vi "Washer HCC Newfi Main.vi"() -> ()   [LabVIEW 2012]
uses:
  Nufi/Newfi LDN/Washer.ctl
  Nufi/Newfi LDN/Washer Details.ctl
  Nufi/Newfi LDN/Unit Type.ctl
  <vilib>/Utility/file.llb/Read From Spreadsheet File (string).vi
  Drivers/Agilent 34970/Agilent 34970.lvlib
panel:
  in  "Tab Control 3":enum32{"Debug Info"}(tab)
  out "Agilent Channels DAQ":string
  out "Current":dbl[](array[numeric])
  out "States Out":string
  out "States Out 2":string
  out "Save Array":bool[](array[boolean])
  out "Board Index.":i32[](array[numeric])
  out "error out":errorcluster
  in  "error in (no error)":errorcluster
  in  "Tab Control 2":enum32{"Page 1"}(tab)
  in  "Quit":bool
  out "Timer 2":dbl format="%<%H:%M:%S>t"
  in  "Connected Board ID's (Newfi)":string[](array[string])
  in  "Board Index":i32[](array[numeric])
  in  "Back Button":bool
  in  "Settings":bool
  out "Description":string="Application Title"
  out "Waveform Chart":dbl(graph)
  in  "Open Panel":T1 {"Unit Type" items=["", "Viper", "Hawk", "Other"]; "Current" format="%.2f"; "Day Cycle Count" format="%04d"}
  in  "Tab Control":enum32{"Page 1", "Page 2"}(tab)
  in  "Array 4":T1[](array[typedef]) {"Unit Type" items=["", "Viper", "Hawk", "Other"]; "Current" format="%.2f"; "Day Cycle Count" format="%04d"}
  in  "Array 3":T1[](array[typedef]) {"Unit Type" items=["", "Viper", "Hawk", "Other"]; "Current" format="%.2f"; "Day Cycle Count" format="%04d"}
  in  "Array":T1[](array[typedef]) {"Unit Type" items=["", "Viper", "Hawk", "Other"]; "Current" format="%.2f"; "Day Cycle Count" format="%04d"}
  in  "Array 2":T1[](array[typedef]) {"Unit Type" items=["", "Viper", "Hawk", "Other"]; "Current" format="%.2f"; "Day Cycle Count" format="%04d"}
  out "Collecting Agilent Data":bool
  in  "Agilent Scan Rate (Seconds)":i32=5
  in  "Status Output Locations":path[](array[path])
  in  "Configuration Path":path=path "C:/Newfi Exe/Newfi Exe Locations.ini"
  out "Time":string="Settings"
  in  "Station and Board IDs":path=path "C:/Newfi Exe/Stations and Board IDs.ini"
  in  "Agilent":refnum<visa-resource-name>="AGILENT_HCC"
  in  "Start DAQ Loop":bool
  # "Washer HCC"
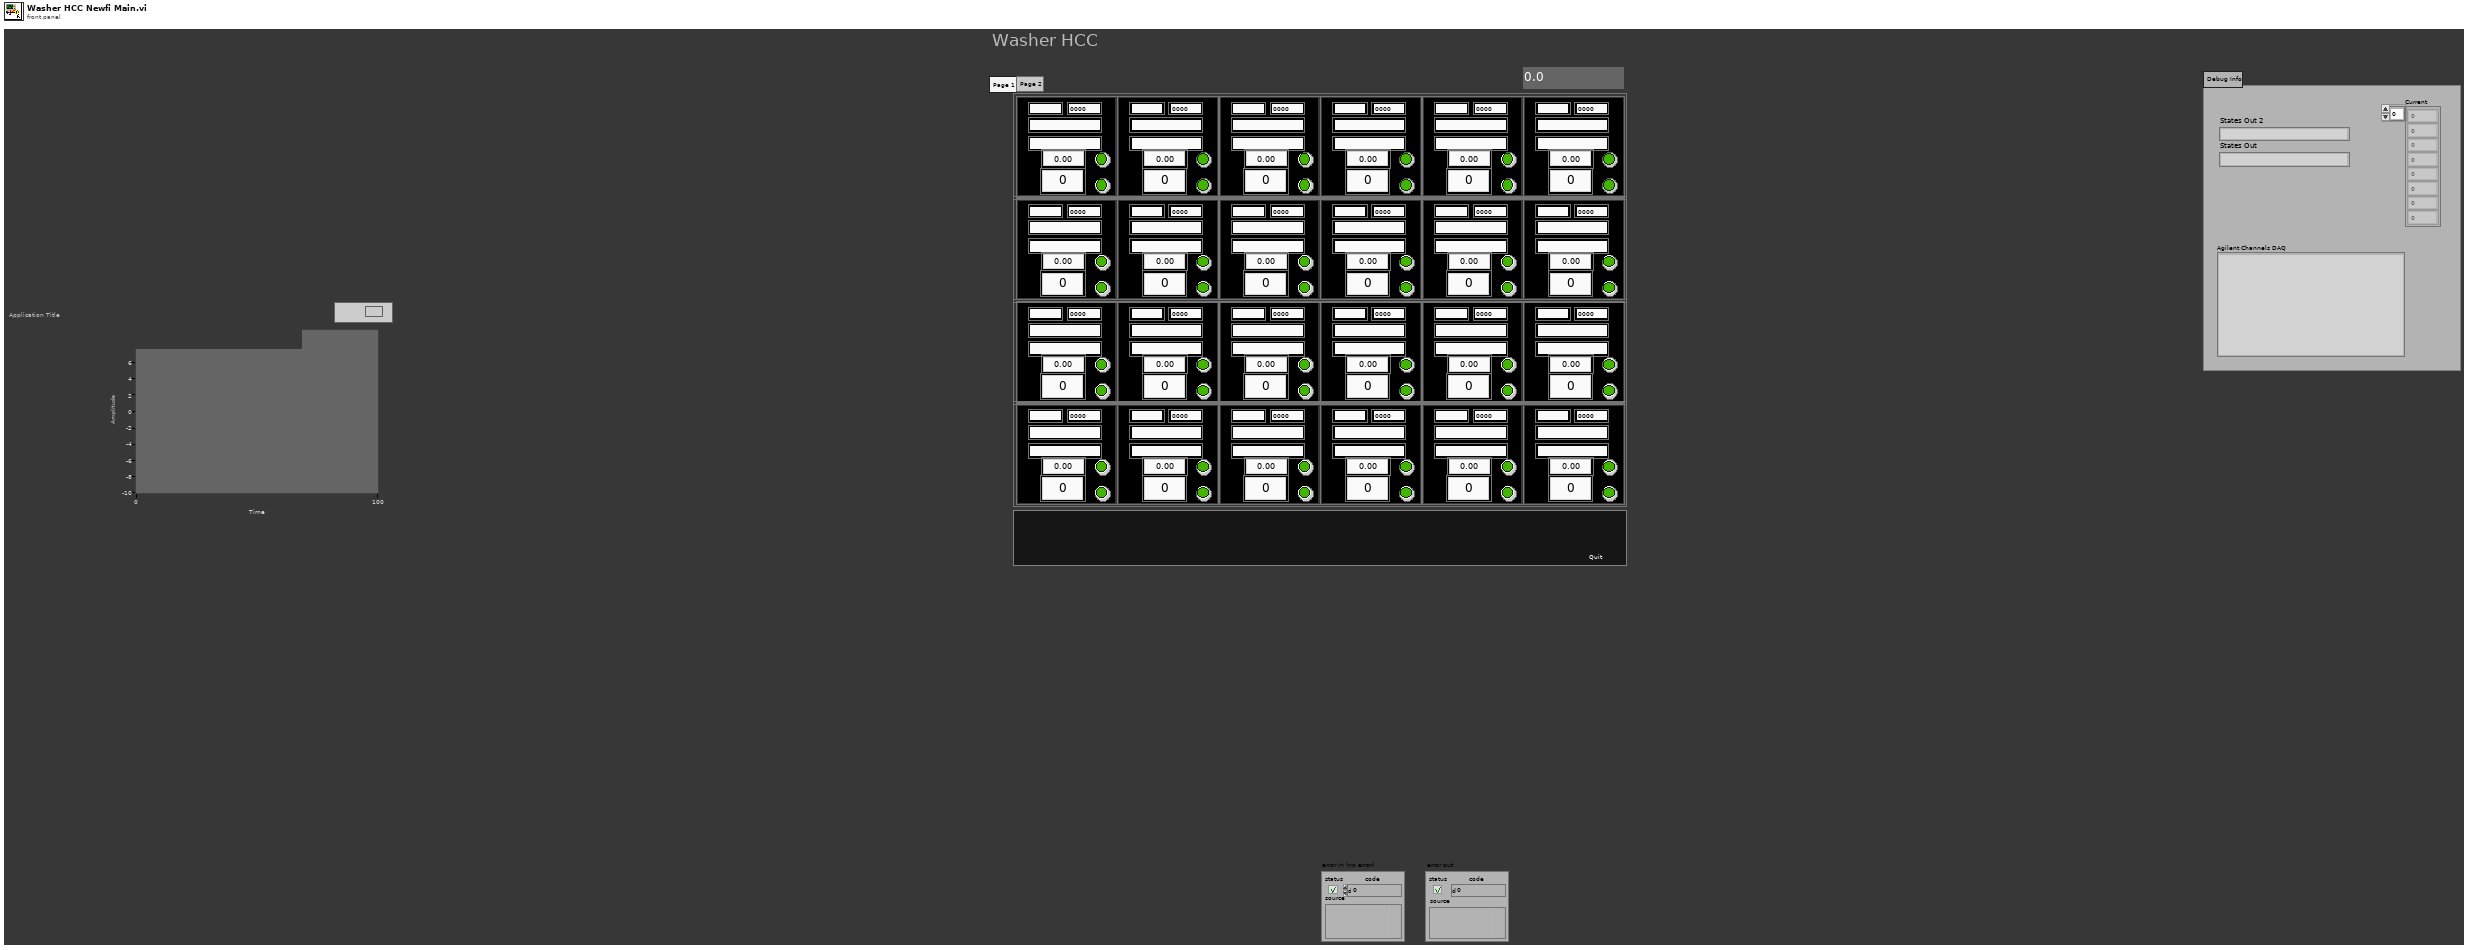
[diagram p1: front panel]
types:
  T1 = typedef "Washer.ctl" = cluster{"Serial Number":string, "Day Cycle Count":i32, "Station Label":string, "Status Color":u32, "Current Run Start Time":dbl, "Audit Alert":bool, "Washer Details":T2, "Board ID":string, "Boolean":bool, "RPM":u32, "Current":dbl, "Current Path":path, "Saving":bool, "Unit Type":T3}
  T2 = typedef "Washer Details.ctl" = cluster{"Cycle Count":string, "Status":string, "Notes":string, "Lab ID":string, "Total Time On":string, "TR Number":string}
  T3 = typedef "Unit Type.ctl" = u32
  T4 = enum16{"4 1/2", "5 1/2", "6 1/2", "Least", "Highest", "Default"}
  T5 = enum16{"100 mV", "1 V", "10 V", "100 V", "300 V", "Auto", "Minimum", "Maximum"}
  T6 = cluster{"Agilent":refnum<visa-resource-name>, "Agilent Scan Rate (Seconds)":i32, "Current":dbl[]}
  T7 = enum32{"invalid app kind", "Development System", "Run Time System", "Student Edition", "Embedded LabVIEW", "Evaluation", "Custom"}
  T8 = cluster{"Current VI Reference":refnum<vi>, "Close Panel on Exit?":bool}
  T9 = enum32{"Invalid", "Standard", "Closed", "Hidden", "Minimized", "Maximized"}
  T10 = cluster{"Core":cluster{"Current VI Reference":refnum<vi>, "Close Panel on Exit?":bool}, "Array":T1[], "Array 2":T1[], "Status Output Locations":path[], "Open Panel":T1, "Array 3":T1[], "Array 4":T1[], "Board Index":i32[], "Connected Board ID's (Newfi)":string[], "Agilent Channels":string, "Start DAQ Loop":bool, "Log Debug":string[], "Log Inv & MC":string[], "Station IDs":string[], "Last Save Time":string}
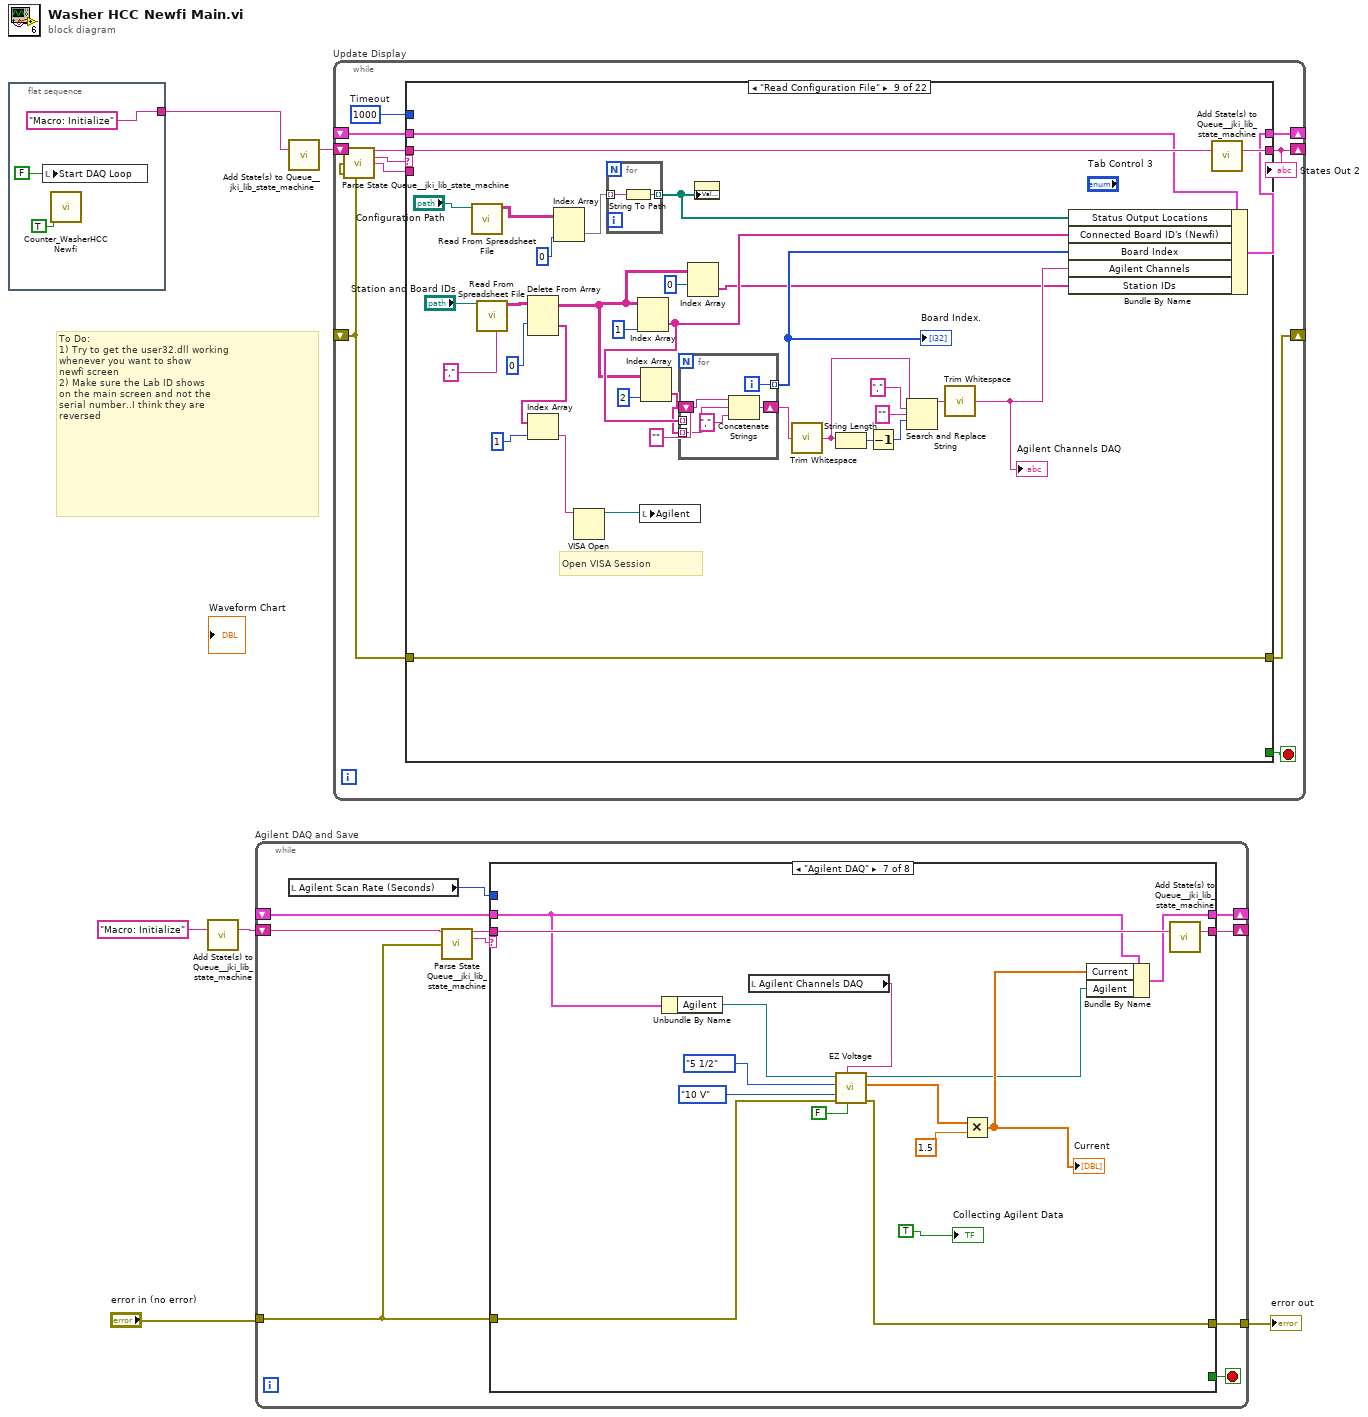
[diagram p0: block diagram]
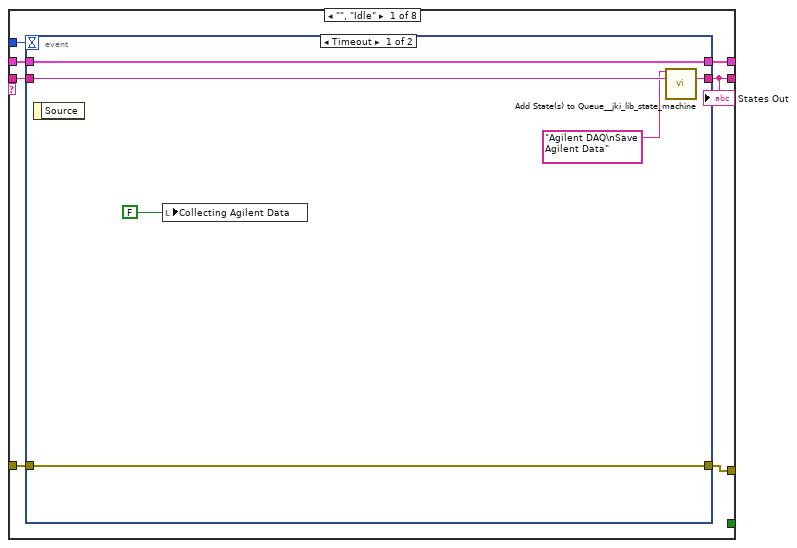
[diagram p2: hidden frame]
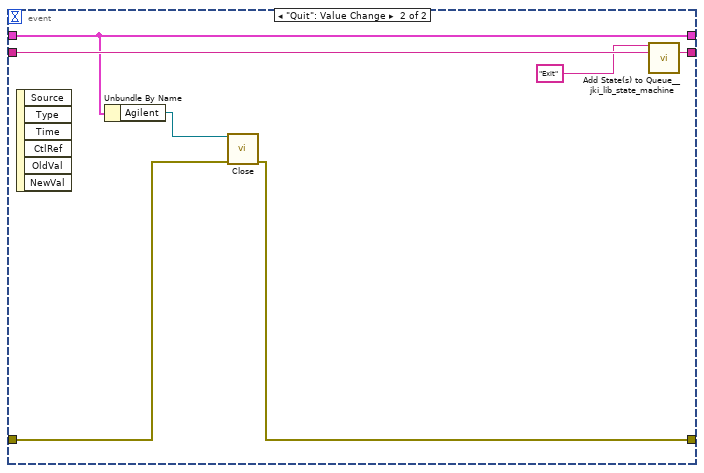
[diagram p3: hidden frame]
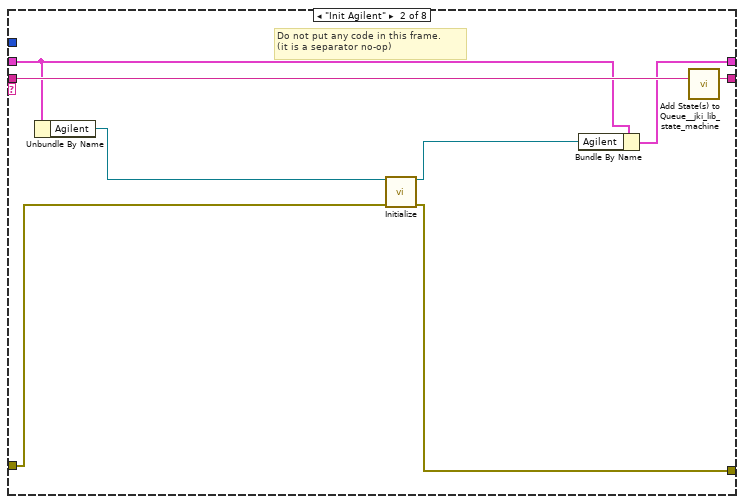
[diagram p4: hidden frame]
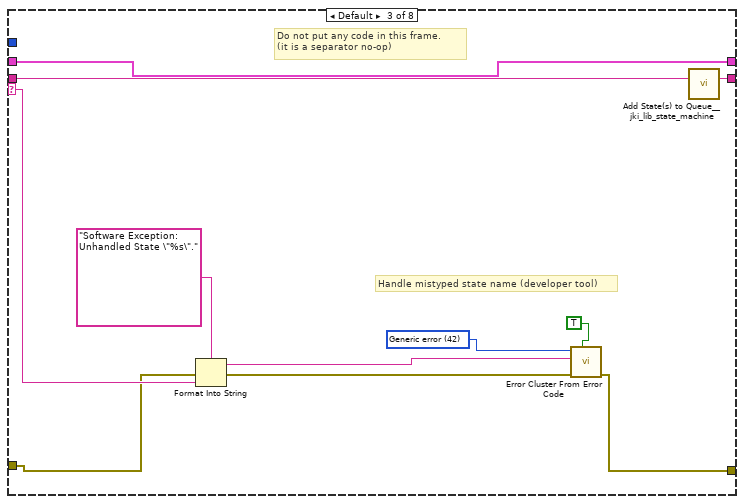
[diagram p5: hidden frame]
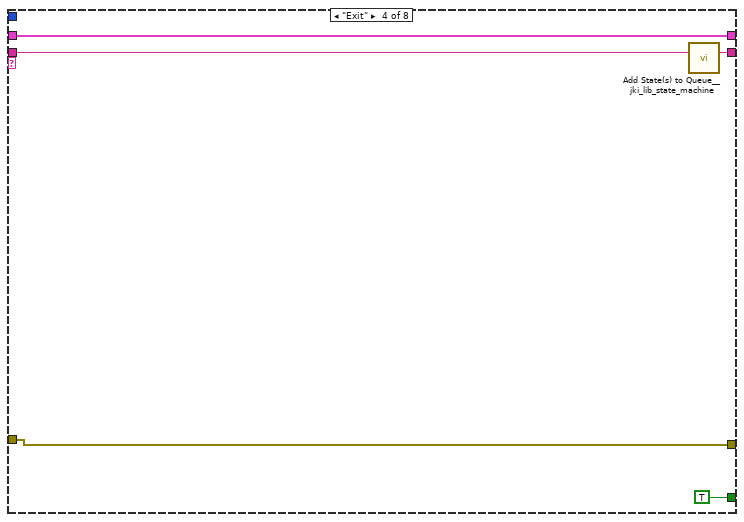
[diagram p6: hidden frame]
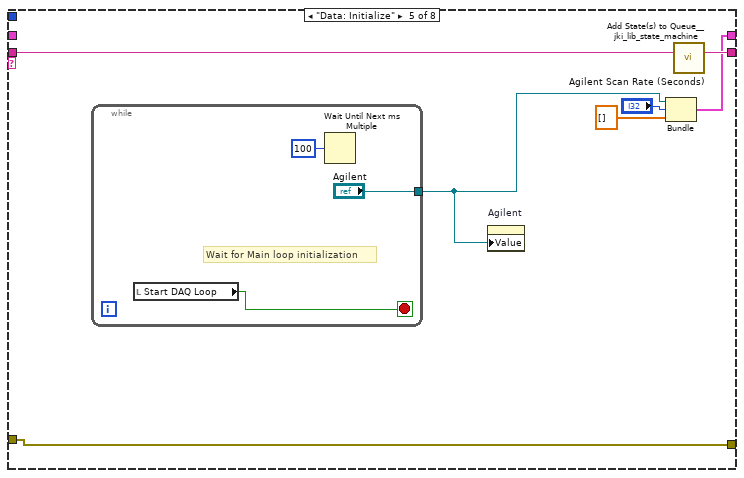
[diagram p7: hidden frame]
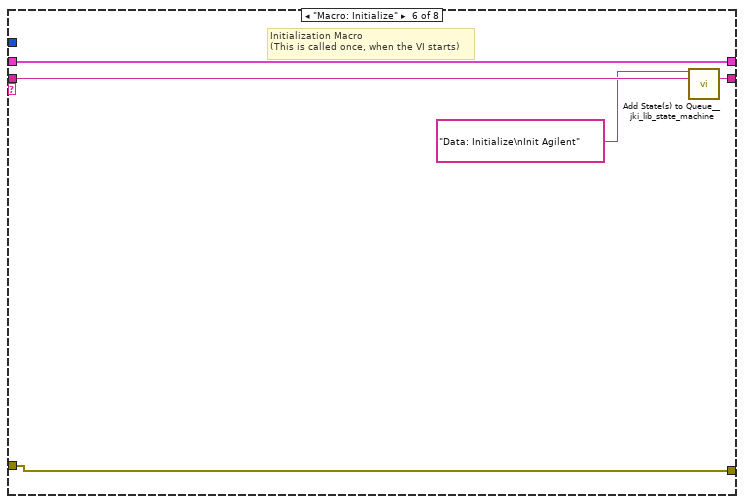
[diagram p8: hidden frame]
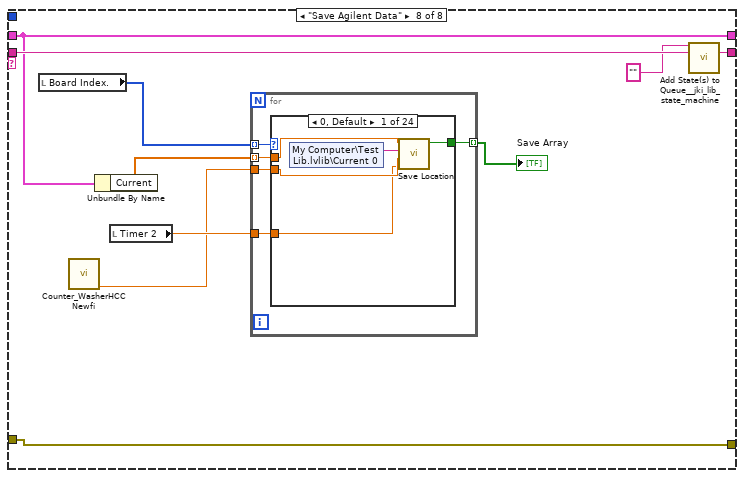
[diagram p9: hidden frame]
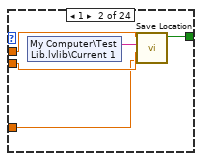
[diagram p10: hidden frame]
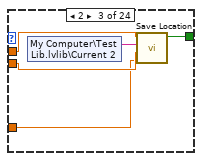
[diagram p11: hidden frame]
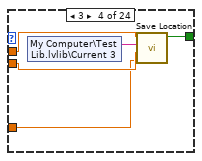
[diagram p12: hidden frame]
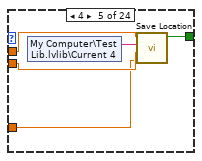
[diagram p13: hidden frame]
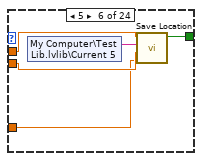
[diagram p14: hidden frame]
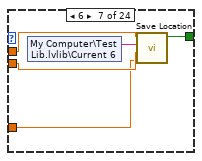
[diagram p15: hidden frame]
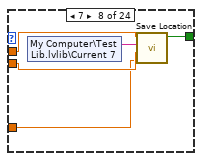
[diagram p16: hidden frame]
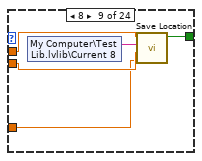
[diagram p17: hidden frame]
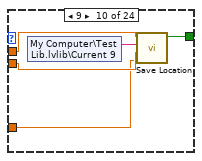
[diagram p18: hidden frame]
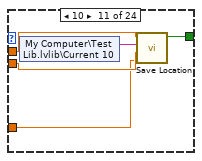
[diagram p19: hidden frame]
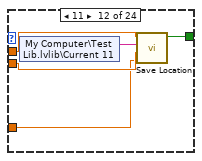
[diagram p20: hidden frame]
diagram:
  # "To Do:\n1) Try to get the user32.dll working\nwhenever you want to show\nnewfi screen\n2) Make sure the Lab ID shows\non the main screen and not the \nserial number..I think they are \nreversed"
  n1 = flat-sequence {
    tunnel: ["Macro: Initialize"] -> w3
    frame #0 {
      n2 = local write "Start DAQ Loop"(FALSE ("Start DAQ Loop")) -> ()
      n3 = call "Counter_WasherHCC Newfi.vi"("Reset"=TRUE) -> ()  [unwired: 10 in, 1 out]
    }
  }
  n4 = call <vilib>:"Add State(s) to Queue__jki_lib_state_machine.vi"("State(s) in (\"\")"="Macro: Initialize") -> ("States Out"=w2:string)  [unwired: 14 in]
  n5 = while "Agilent DAQ and Save" {
    shift-right: [w14] -> _
    shift-left: _ -> [w13]
    shift-right: [w16] -> _
    shift-left: w2 -> [w17]
    tunnel: "error in (no error)" -> [w10]
    tunnel: [w12] -> w5
    stop <- w15 stop-if-true
    n6 = local read "Agilent Scan Rate (Seconds)"() -> (w11:i32)
    n7 = call <vilib>:"Parse State Queue__jki_lib_state_machine.vi"("State Queue"=w17, "Error In (no error)"=w10) -> ("Remaining States"=w18:string, "Current State"=w19:string)  [unwired: 11 in, 1 out]
    n8 = case shown="\"Agilent DAQ\"" w19 {
      selector: w19 -> [_ _ w50 _ _ _ _ _]
      tunnel: w18 -> [w26 w47 w58 w63 w70 w78 w94 w104]
      tunnel: w13 -> [w24 w44 w56 w61 _ w76 w84 w98]
      tunnel: [w25 w46 w57 w62 w69 w77 w93 w103] -> w16
      tunnel: [_ _ _ TRUE _ _ _ _] -> w15
      tunnel: [w23 w43 w56 w61 w68 w76 w83 w98] -> w14
      tunnel: w11 -> [w22 _ _ _ _ _ _ _]
      tunnel: w10 -> [w21 w41 w49 w59 w65 w74 w86 w102]
      tunnel: [w20 w40 w48 w59 w65 w74 w85 w102] -> w12
      frame "", "Idle" {
        n9 = event shown="[0] Timeout" {
          selector: _ -> [_ _]
          dyn-events: _ -> [_ _]
          timeout: w22 -> [_ _]
          tunnel: w26 -> [w32 w39]
          tunnel: [w31 w38] -> w25
          tunnel: w24 -> [w30 w36]
          tunnel: [w30 w36] -> w23
          tunnel: [w27 w33] -> w20
          tunnel: w21 -> [w27 w34]
          event Timeout {
            n10 = event-data() -> ()  [unwired: 1 in, 1 out]
            n11 = local write "Collecting Agilent Data"(FALSE ("Collecting Agilent Data")) -> ()
            n12 = call <vilib>:"Add State(s) to Queue__jki_lib_state_machine.vi"("State(s) in Front (\"\")"="Agilent DAQ\nSave Agilent Data", "State(s) in (\"\")"=w32) -> ("States Out"=w31:string)  [unwired: 13 in]
          }
          event "Quit": Value Change {
            n13 = event-data() -> ()  [unwired: 1 in, 6 out]
            n14 = Unbundle By Name(w36) -> ("Agilent"=w35:refnum<visa-resource-name>)
            n15 = call "Close.vi"("VISA Resource Name"=w35, "error in (no error)"=w34) -> ("error out"=w33:errorcluster)  [unwired: 13 in]
            n16 = call <vilib>:"Add State(s) to Queue__jki_lib_state_machine.vi"("State(s) in Front (\"\")"="Exit", "State(s) in (\"\")"=w39) -> ("States Out"=w38:string)  [unwired: 13 in]
          }
        }
        "States Out" <- w25
      }
      frame "Init Agilent" {
        # "Do not put any code in this frame.\n(it is a separator no-op)"
        n17 = Unbundle By Name(w44) -> ("Agilent"=w45:refnum<visa-resource-name>)
        n18 = call "Initialize.vi"("VISA Resource Name"=w45, "error in (no error)"=w41) -> ("VISA Resource Name Out"=w42:refnum<visa-resource-name>, "error out"=w40:errorcluster)  [unwired: 12 in]
        n19 = Bundle By Name(cluster=w44, "Agilent"=w42) -> (w43:T6)
        n20 = call <vilib>:"Add State(s) to Queue__jki_lib_state_machine.vi"("State(s) in (\"\")"=w47) -> ("States Out"=w46:string)  [unwired: 14 in]
      }
      frame Default {
        w52 = 42 items=["No error", "Argument error", "Memory is full", "Out of zone", "End of file", "File already open", "Generic file I/O error", "File not found", "File permission error", "Disk is full", "Duplicate path", "Too many files open", "System feature not enabled", "Resource file not found", "Cannot add resource", "Resource not found", "Image not found", "Image memory error", "Pen does not exist", "Config type invalid", "Config token not found", "Config parse error", "Config memory error", "Bad external code format", "Bad external code offset", "External code not present", "Null window", "Destroy window error", "Null menu", "Print aborted", "Bad print record", "Print driver error", "Windows error during printing", "Memory error during printing", "Print dialog error", "Generic print error", "Invalid device refnum", "Device not found", "Device parameter error", "Device unit error", "Cannot open device", "Device call aborted", "Generic error", "Cancelled by user", "Object ID too low", "Object ID too high", "Object not in heap", "Unknown heap", "Unknown object (invalid DefProc)", "Unknown object (DefProc not in table)", "Message out of range", "Invalid (null) method", "Unknown message", "Manager call not supported", "Bad address", "Network operation in progress", "Network operation timed out", "Connection is busy", "Network attribute not supported", "Network error", "Address in use", "System out of memory", "Connection aborted", "Connection refused", "Not connected", "Already connected", "Connection closed", "Initialization error (interapplication manager)", "Bad occurrence", "Wait on unbound occurrence handler", "Occurrence queue overflow", "Datalog type conflict", "Unused", "Unrecognized type (interapplication manager)", "Memory corrupt", "Failed to make temporary DLL", "Old CIN version", "Drag socket not found", "Failed to load drop-object", "Failed to register OLE object", "Failed to release OLE object", "Format specifier type mismatch", "Unknown format specifier", "Too few format specifiers", "Too many format specifiers", "Scan failed", "Newer CIN version", "Error converting to variant", "Runtime menu error", "Password tampered", "Variant attribute not found", "Incompatible variant data type", "Event data is not available", "Event Store is not present", "Occurrence is not found", "Event Queue is not created", "Event info is not available", "Refnum passed is NULL", "Error retrieving Class GUID", "Error retrieving CoClass GUID", "Error retrieving TypeLib GUID.", "Bad built application magic bytes.", "Specific driver is different from the specific driver associated with the Logical Name.", "There is no session opened to the class driver.", "Max Error", "MAX - Error with config objects", "MAX - Error loading configuration", "MAX - Group not supported"]
        # "Handle mistyped state name (developer tool)"
        # "Do not put any code in this frame.\n(it is a separator no-op)"
        n21 = Format Into String(format string="Software Exception: Unhandled State \"%s\"." ("message"), error in=w49, w50) -> (resulting string=w53:string, error out=w54:errorcluster)  [unwired: 1 in]
        n22 = call <vilib>:"Error Cluster From Error Code.vi"("show call chain? (False)"=TRUE, "error in (no error)"=w54, "error message (\"\")"=w53, "error code (0)"=w52) -> ("error out"=w48:errorcluster)  [unwired: 5 in]
        n23 = call <vilib>:"Add State(s) to Queue__jki_lib_state_machine.vi"("State(s) in (\"\")"=w58) -> ("States Out"=w57:string)  [unwired: 14 in]
      }
      frame "Exit" {
        n24 = call <vilib>:"Add State(s) to Queue__jki_lib_state_machine.vi"("State(s) in (\"\")"=w63) -> ("States Out"=w62:string)  [unwired: 14 in]
      }
      frame "Data: Initialize" {
        n25 = while {
          tunnel: ["Agilent"] -> w64
          stop <- w72 stop-if-true
          # "Wait for Main loop initialization"
          n26 = local read "Start DAQ Loop"() -> (w72:bool)
          n27 = Wait Until Next ms Multiple(millisecond multiple=u32 100) -> ()  [unwired: 1 out]
        }
        n28 = property on="Agilent" class="VISAName"("Value"=w64) -> ()  [unwired: 2 in, 2 out]
        n29 = Bundle("Agilent"=w64, "Agilent Scan Rate (Seconds)"="Agilent Scan Rate (Seconds)", "Current"=dbl[] []) -> (w68:T6)  [unwired: 1 in]
        n30 = call <vilib>:"Add State(s) to Queue__jki_lib_state_machine.vi"("State(s) in (\"\")"=w70) -> ("States Out"=w69:string)  [unwired: 14 in]
      }
      frame "Macro: Initialize" {
        # "Initialization Macro\n(This is called once, when the VI starts)"
        n31 = call <vilib>:"Add State(s) to Queue__jki_lib_state_machine.vi"("State(s) in Front (\"\")"="Data: Initialize\nInit Agilent", "State(s) in (\"\")"=w78) -> ("States Out"=w77:string)  [unwired: 13 in]
      }
      frame "Agilent DAQ" {
        n32 = Unbundle By Name(w84) -> ("Agilent"=w92:refnum<visa-resource-name>)
        n33 = local read "Agilent Channels DAQ"() -> (w81:string)
        n34 = call "EZ Voltage.vi"("AC/DC (F:DC)"=FALSE, "Scan List (empty)"=w81, "error in (no error)"=w86, "Range (5:Auto)"=T5."10 V", "Resolution (5:Default)"=T4."5 1/2", "VISA Resource Name"=w92) -> ("error out"=w85:errorcluster, "Output Array"=w88:dbl[], "VISA Resource Name Out"=w79:refnum<visa-resource-name>)  [unwired: 3 in]
        n35 = Multiply(x=w88, y=1.5) -> (x*y=w80:dbl[])
        "Current" <- w80
        n36 = Bundle By Name(cluster=w84, "Current"=w80, "Agilent"=w79) -> (w83:T6)
        n37 = call <vilib>:"Add State(s) to Queue__jki_lib_state_machine.vi"("State(s) in (\"\")"=w94) -> ("States Out"=w93:string)  [unwired: 14 in]
        "Collecting Agilent Data" <- TRUE
      }
      frame "Save Agilent Data" {
        n38 = local read "Board Index."() -> (w99:i32[])
        n39 = call "Counter_WasherHCC Newfi.vi"() -> ("Count"=w96:dbl)  [unwired: 11 in]
        n40 = Unbundle By Name(w98) -> ("Current"=w101:dbl[])
        n41 = local read "Timer 2"() -> (w97:dbl)
        n42 = for {
          tunnel: w99 -> [w109] mode=indexing
          tunnel: w101 -> [w108] mode=indexing
          tunnel: w96 -> [w107]
          tunnel: [w106] -> w100 mode=indexing
          tunnel: w97 -> [w105]
          n43 = case shown="0, Default" w109 {
            tunnel: w108 -> [w113 w118 w123 w128 w133 w138 w143 w149 w153 w158 w164 w168 w174 w178 w183 w188 w193 w198 w203 w208 w213 w218 w224 w226]
            tunnel: w107 -> [w112 w117 w122 w127 w132 w137 w142 w147 w152 w157 w162 w167 w172 w177 w182 w187 w192 w197 w202 w207 w212 w217 w222 w228]
            tunnel: [w111 w116 w121 w126 w131 w136 w141 w146 w151 w156 w161 w166 w171 w176 w181 w186 w191 w196 w201 w206 w211 w216 w221 w227] -> w106
            tunnel: w105 -> [w110 w115 w120 w125 w130 w135 w140 w145 w150 w155 w160 w165 w170 w175 w180 w185 w190 w195 w200 w205 w210 w215 w220 w225]
            frame 0, Default {
              n44 = shared-variable "My Computer\\Test Lib.lvlib\\Current 0"() -> (w114:string)  [unwired: 1 in, 1 out]
              n45 = call "Save Location.vi"("Timer Seconds"=w110, "Counter"=w112, "String"=w114, "Current"=w113) -> ("Saving"=w111:bool)  [unwired: 7 in]
            }
            frame 1 {
              n46 = shared-variable "My Computer\\Test Lib.lvlib\\Current 1"() -> (w119:string)  [unwired: 1 in, 1 out]
              n47 = call "Save Location.vi"("Timer Seconds"=w115, "Counter"=w117, "String"=w119, "Current"=w118) -> ("Saving"=w116:bool)  [unwired: 7 in]
            }
            frame 2 {
              n48 = shared-variable "My Computer\\Test Lib.lvlib\\Current 2"() -> (w124:string)  [unwired: 1 in, 1 out]
              n49 = call "Save Location.vi"("Timer Seconds"=w120, "Counter"=w122, "String"=w124, "Current"=w123) -> ("Saving"=w121:bool)  [unwired: 7 in]
            }
            frame 3 {
              n50 = shared-variable "My Computer\\Test Lib.lvlib\\Current 3"() -> (w129:string)  [unwired: 1 in, 1 out]
              n51 = call "Save Location.vi"("Timer Seconds"=w125, "Counter"=w127, "String"=w129, "Current"=w128) -> ("Saving"=w126:bool)  [unwired: 7 in]
            }
            frame 4 {
              n52 = shared-variable "My Computer\\Test Lib.lvlib\\Current 4"() -> (w134:string)  [unwired: 1 in, 1 out]
              n53 = call "Save Location.vi"("Timer Seconds"=w130, "Counter"=w132, "String"=w134, "Current"=w133) -> ("Saving"=w131:bool)  [unwired: 7 in]
            }
            frame 5 {
              n54 = shared-variable "My Computer\\Test Lib.lvlib\\Current 5"() -> (w139:string)  [unwired: 1 in, 1 out]
              n55 = call "Save Location.vi"("Timer Seconds"=w135, "Counter"=w137, "String"=w139, "Current"=w138) -> ("Saving"=w136:bool)  [unwired: 7 in]
            }
            frame 6 {
              n56 = shared-variable "My Computer\\Test Lib.lvlib\\Current 6"() -> (w144:string)  [unwired: 1 in, 1 out]
              n57 = call "Save Location.vi"("Timer Seconds"=w140, "Counter"=w142, "String"=w144, "Current"=w143) -> ("Saving"=w141:bool)  [unwired: 7 in]
            }
            frame 7 {
              n58 = shared-variable "My Computer\\Test Lib.lvlib\\Current 7"() -> (w148:string)  [unwired: 1 in, 1 out]
              n59 = call "Save Location.vi"("Timer Seconds"=w145, "Counter"=w147, "String"=w148, "Current"=w149) -> ("Saving"=w146:bool)  [unwired: 7 in]
            }
            frame 8 {
              n60 = shared-variable "My Computer\\Test Lib.lvlib\\Current 8"() -> (w154:string)  [unwired: 1 in, 1 out]
              n61 = call "Save Location.vi"("Timer Seconds"=w150, "Counter"=w152, "String"=w154, "Current"=w153) -> ("Saving"=w151:bool)  [unwired: 7 in]
            }
            frame 9 {
              n62 = shared-variable "My Computer\\Test Lib.lvlib\\Current 9"() -> (w159:string)  [unwired: 1 in, 1 out]
              n63 = call "Save Location.vi"("Timer Seconds"=w155, "Counter"=w157, "String"=w159, "Current"=w158) -> ("Saving"=w156:bool)  [unwired: 7 in]
            }
            frame 10 {
              n64 = shared-variable "My Computer\\Test Lib.lvlib\\Current 10"() -> (w163:string)  [unwired: 1 in, 1 out]
              n65 = call "Save Location.vi"("Timer Seconds"=w160, "Counter"=w162, "String"=w163, "Current"=w164) -> ("Saving"=w161:bool)  [unwired: 7 in]
            }
            frame 11 {
              n66 = shared-variable "My Computer\\Test Lib.lvlib\\Current 11"() -> (w169:string)  [unwired: 1 in, 1 out]
              n67 = call "Save Location.vi"("Timer Seconds"=w165, "Counter"=w167, "String"=w169, "Current"=w168) -> ("Saving"=w166:bool)  [unwired: 7 in]
            }
            frame 12 {
              n68 = shared-variable "My Computer\\Test Lib.lvlib\\Current 12"() -> (w173:string)  [unwired: 1 in, 1 out]
              n69 = call "Save Location.vi"("Timer Seconds"=w170, "Counter"=w172, "String"=w173, "Current"=w174) -> ("Saving"=w171:bool)  [unwired: 7 in]
            }
            frame 13 {
              n70 = shared-variable "My Computer\\Test Lib.lvlib\\Current 13"() -> (w179:string)  [unwired: 1 in, 1 out]
              n71 = call "Save Location.vi"("Timer Seconds"=w175, "Counter"=w177, "String"=w179, "Current"=w178) -> ("Saving"=w176:bool)  [unwired: 7 in]
            }
            frame 14 {
              n72 = shared-variable "My Computer\\Test Lib.lvlib\\Current 14"() -> (w184:string)  [unwired: 1 in, 1 out]
              n73 = call "Save Location.vi"("Timer Seconds"=w180, "Counter"=w182, "String"=w184, "Current"=w183) -> ("Saving"=w181:bool)  [unwired: 7 in]
            }
            frame 15 {
              n74 = shared-variable "My Computer\\Test Lib.lvlib\\Current 15"() -> (w189:string)  [unwired: 1 in, 1 out]
              n75 = call "Save Location.vi"("Timer Seconds"=w185, "Counter"=w187, "String"=w189, "Current"=w188) -> ("Saving"=w186:bool)  [unwired: 7 in]
            }
            frame 16 {
              n76 = shared-variable "My Computer\\Test Lib.lvlib\\Current 16"() -> (w194:string)  [unwired: 1 in, 1 out]
              n77 = call "Save Location.vi"("Timer Seconds"=w190, "Counter"=w192, "String"=w194, "Current"=w193) -> ("Saving"=w191:bool)  [unwired: 7 in]
            }
            frame 17 {
              n78 = shared-variable "My Computer\\Test Lib.lvlib\\Current 17"() -> (w199:string)  [unwired: 1 in, 1 out]
              n79 = call "Save Location.vi"("Timer Seconds"=w195, "Counter"=w197, "String"=w199, "Current"=w198) -> ("Saving"=w196:bool)  [unwired: 7 in]
            }
            frame 18 {
              n80 = shared-variable "My Computer\\Test Lib.lvlib\\Current 18"() -> (w204:string)  [unwired: 1 in, 1 out]
              n81 = call "Save Location.vi"("Timer Seconds"=w200, "Counter"=w202, "String"=w204, "Current"=w203) -> ("Saving"=w201:bool)  [unwired: 7 in]
            }
            frame 19 {
              n82 = shared-variable "My Computer\\Test Lib.lvlib\\Current 19"() -> (w209:string)  [unwired: 1 in, 1 out]
              n83 = call "Save Location.vi"("Timer Seconds"=w205, "Counter"=w207, "String"=w209, "Current"=w208) -> ("Saving"=w206:bool)  [unwired: 7 in]
            }
            frame 20 {
              n84 = shared-variable "My Computer\\Test Lib.lvlib\\Current 20"() -> (w214:string)  [unwired: 1 in, 1 out]
              n85 = call "Save Location.vi"("Timer Seconds"=w210, "Counter"=w212, "String"=w214, "Current"=w213) -> ("Saving"=w211:bool)  [unwired: 7 in]
            }
            frame 21 {
              n86 = shared-variable "My Computer\\Test Lib.lvlib\\Current 21"() -> (w219:string)  [unwired: 1 in, 1 out]
              n87 = call "Save Location.vi"("Timer Seconds"=w215, "Counter"=w217, "String"=w219, "Current"=w218) -> ("Saving"=w216:bool)  [unwired: 7 in]
            }
            frame 22 {
              n88 = shared-variable "My Computer\\Test Lib.lvlib\\Current 22"() -> (w223:string)  [unwired: 1 in, 1 out]
              n89 = call "Save Location.vi"("Timer Seconds"=w220, "Counter"=w222, "String"=w223, "Current"=w224) -> ("Saving"=w221:bool)  [unwired: 7 in]
            }
            frame 23 {
              n90 = shared-variable "My Computer\\Test Lib.lvlib\\Current 23"() -> (w229:string)  [unwired: 1 in, 1 out]
              n91 = call "Save Location.vi"("Timer Seconds"=w225, "Counter"=w228, "String"=w229, "Current"=w226) -> ("Saving"=w227:bool)  [unwired: 7 in]
            }
          }
        }
        "Save Array" <- w100
        n92 = call <vilib>:"Add State(s) to Queue__jki_lib_state_machine.vi"("State(s) in Front (\"\")"="" ("State(s) in Front (\"\")"), "State(s) in (\"\")"=w104) -> ("States Out"=w103:string)  [unwired: 13 in]
      }
    }
  }
  "error out" <- w5
  n93 = call <vilib>:"Add State(s) to Queue__jki_lib_state_machine.vi"("State(s) in (\"\")"=w3) -> ("States Out"=w6:string)  [unwired: 14 in]
  n94 = while "Update Display" {
    shift-right: [w233] -> _
    shift-left: _ -> [w232]
    shift-right: [w236] -> _
    shift-left: _ -> [w230]
    shift-right: [w235] -> _
    shift-left: w6 -> [w237]
    stop <- w234 stop-if-true
    w231 = 1000  # Timeout
    n95 = call <vilib>:"Parse State Queue__jki_lib_state_machine.vi"("State Queue"=w237, "Error In (no error)"=w230) -> ("Remaining States"=w239:string, "Current State"=w240:string, "Arguments"=w238:string)  [unwired: 11 in]
    n96 = case shown="\"Read Configuration File\"" w240 {
      selector: w240 -> [_ _ w439 _ _ _ _ _ _ _ _ _ _ _ _ _ _ _ _ _ _ _]
      tunnel: w239 -> [w247 w438 w443 w461 w467 w472 w476 w495 w526 w558 w577 w581 w587 w593 w605 w631 w636 w646 w650 w686 w691 w695]
      tunnel: w238 -> [_ _ _ _ _ _ _ _ _ _ _ _ _ w588 w599 _ _ _ _ _ _ _]
      tunnel: w232 -> [w245 w435 w441 w452 w464 w470 w473 _ w525 w543 w572 w578 w584 w591 w601 w628 w633 w643 w647 w683 w689 w693]
      tunnel: [w244 w436 w445 w458 errorcluster {"status"=FALSE, "code"=0, "source"=""} ("error out") w469 w474 w492 w522 w557 w573 w579 w585 w589 w602 w629 w634 w644 w648 w684 w688 w692] -> w236
      tunnel: w230 -> [w243 w436 w444 w458 w463 w469 w474 w492 w522 w557 w574 w579 w585 w590 w603 w629 w634 w644 w648 w684 w688 w692]
      tunnel: [w246 w437 w442 w460 w466 w471 w475 w494 w530 w559 w576 w580 w586 w592 w604 w630 w635 w645 w649 w685 w690 w694] -> w235
      tunnel: [_ _ _ _ _ TRUE _ _ _ _ _ _ _ _ _ _ _ _ _ _ _ _] -> w234
      tunnel: [w242 w435 w441 w459 w464 w470 w473 w493 w524 w542 w572 w578 w583 w591 w601 w628 w633 w643 w647 w682 w689 w693] -> w233
      tunnel: w231 -> [w241 _ _ _ _ _ _ _ _ _ _ _ _ _ _ _ _ _ _ _ _ _]
      frame "", "Idle" {
        n97 = event shown="[0] Timeout" {
          selector: _ -> [_ _ _ _ _ _ _ _ _]
          dyn-events: _ -> [_ _ _ _ _ _ _ _ _]
          timeout: w241 -> [_ _ _ _ _ _ _ _ _]
          tunnel: w247 -> [w253 w259 w274 w317 w356 w395 w421 w426 w434]
          tunnel: [w252 w258 w273 w316 w355 w394 w421 w426 w433] -> w246
          tunnel: w245 -> [w250 w257 w269 w307 w346 w385 w422 w425 w431]
          tunnel: [w251 w254 w264 w318 w357 w396 w423 w427 w432] -> w244
          tunnel: w243 -> [w251 w254 w265 w318 w357 w396 w423 w427 w432]
          tunnel: [w250 w257 w272 w314 w353 w392 w422 w425 w431] -> w242
          event Timeout {
            n98 = event-data() -> ()  [unwired: 1 in, 1 out]
            n99 = call "E-Time LDN.vi"() -> ("Elapsed Time (sec)"=→"Timer 2":dbl)  [unwired: 9 in, 2 out]
            n100 = call <vilib>:"Add State(s) to Queue__jki_lib_state_machine.vi"("State(s) in Front (\"\")"="Update Status", "State(s) in (\"\")"=w253) -> ("States Out"=w252:string)  [unwired: 13 in]
          }
          event "Quit": Value Change {
            n101 = event-data() -> ()  [unwired: 1 in, 1 out]
            n102 = shared-variable "My Computer\\Test Lib.lvlib\\Exit"("Quit") -> ()  [unwired: 1 in, 1 out]
            n103 = call <vilib>:"Add State(s) to Queue__jki_lib_state_machine.vi"("State(s) in Front (\"\")"="Macro: Exit", "State(s) in (\"\")"=w259) -> ("States Out"=w258:string)  [unwired: 13 in]
          }
          event "Array": Value Change {
            n104 = event-data() -> ("NewVal"=w263:T1[])  [unwired: 1 in, 5 out]
            n105 = Unbundle By Name(w269) -> ("Open Panel"=w268:T1, "Status Output Locations"=w261:path[], "Connected Board ID's (Newfi)"=w260:string[])
            n106 = for {
              tunnel: w263 -> [w303] mode=indexing
              tunnel: [w301] -> w266
              tunnel: [w299] -> w270 mode=indexing
              i -> [w301]
              stop <- w300 stop-if-true
              n107 = Unbundle By Name(w303) -> ("Boolean"=w299:bool)
              n108 = Equal?(x=w299, y=TRUE) -> (x = y?=w300:bool)
            }
            n109 = Or Array Elements(Boolean array=w270) -> (logical OR=w267:bool)
            n110 = case shown="True" w267 {
              tunnel: w263 -> [_ w285]
              tunnel: w266 -> [_ w279]
              tunnel: [w276 w280] -> w271
              tunnel: w268 -> [w276 _]
              tunnel: w261 -> [_ w284]
              tunnel: w265 -> [w275 w283]
              tunnel: [w275 w282] -> w264
              tunnel: w260 -> [_ w278]
              frame False {
              }
              frame True {
                n111 = disable-structure shown="Enabled" {
                  disable-tunnel: w279 -> [w291 _]
                  disable-tunnel: w284 -> [w290 _]
                  disable-tunnel: w283 -> [w289 _]
                  disable-tunnel: [w287 _] -> w282
                  frame Enabled {
                    n112 = Index Array(array=w290, index=w291) -> (element=w298:path)
                    n113 = Strip Path(path=w298) -> (stripped path=w292:path)  [unwired: 1 out]
                    n114 = Strip Path(path=w292) -> (stripped path=w293:path)  [unwired: 1 out]
                    n115 = Build Path(base path=w293, name or relative path="Newfi.exe") -> (appended path=w295:path)
                    n116 = Path To String(path=w295) -> (string=w296:string)
                    n117 = call <vilib>:"System Exec.vi"("wait until completion? (T)"=FALSE, "error in (no error)"=w289, "command line"=w296) -> ("error out"=w288:errorcluster)  [unwired: 5 in, 3 out]
                    n118 = call "Delay mS.vi"("Error In"=w288, "milliseconds to wait"=u32 2000) -> ("Error Out"=w287:errorcluster)  [unwired: 13 in]
                  }
                  frame Disabled {
                  }
                }
                n119 = Index Array(array=w285, index=w279) -> (element=w281:T1)
                n120 = Index Array(array=w278, index=w279) -> (element=w277:string)
                n121 = Bundle By Name(cluster=w281, "Board ID"=w277) -> (w280:T1)
              }
            }
            n122 = Bundle By Name(cluster=w269, "Open Panel"=w271) -> (w272:T10)
            n123 = call <vilib>:"Add State(s) to Queue__jki_lib_state_machine.vi"("State(s) in Front (\"\")"="Open Newfi Panel", "State(s) in (\"\")"=w274) -> ("States Out"=w273:string)  [unwired: 13 in]
          }
          event "Array 2": Value Change {
            # "Row 7-12"
            n124 = event-data() -> ("NewVal"=w305:T1[])  [unwired: 1 in, 5 out]
            n125 = for {
              tunnel: w305 -> [w342] mode=indexing
              tunnel: [w339] -> w309
              tunnel: [w338] -> w311 mode=indexing
              i -> [w339]
              stop <- w340 stop-if-true
              n126 = Unbundle By Name(w342) -> ("Boolean"=w338:bool)
              n127 = Equal?(x=w338, y=TRUE) -> (x = y?=w340:bool)
            }
            n128 = Unbundle By Name(w307) -> ("Open Panel"=w312:T1, "Status Output Locations"=w308:path[], "Connected Board ID's (Newfi)"=w306:string[])
            n129 = Or Array Elements(Boolean array=w311) -> (logical OR=w310:bool)
            n130 = case shown="True" w310 {
              tunnel: w305 -> [_ w328]
              tunnel: w309 -> [_ w322]
              tunnel: [w319 w324] -> w313
              tunnel: w312 -> [w319 _]
              tunnel: w308 -> [_ w327]
              tunnel: w306 -> [_ w326]
              tunnel: 6 ("size(s)") -> [_ w321]
              frame False {
              }
              frame True {
                n131 = Add(x=w322, y=w321) -> (x+y=w320:i32)
                n132 = disable-structure shown="Enabled" {
                  disable-tunnel: w320 -> [w330 _]
                  disable-tunnel: w327 -> [w329 _]
                  frame Enabled {
                    n133 = Index Array(array=w329, index=w330) -> (element=w331:path)
                    n134 = Strip Path(path=w331) -> (stripped path=w337:path)  [unwired: 1 out]
                    n135 = Strip Path(path=w337) -> (stripped path=w336:path)  [unwired: 1 out]
                    n136 = Build Path(base path=w336, name or relative path="Newfi.exe") -> (appended path=w334:path)
                    n137 = Path To String(path=w334) -> (string=w333:string)
                    n138 = call <vilib>:"System Exec.vi"("wait until completion? (T)"=FALSE, "command line"=w333) -> ()  [unwired: 6 in, 4 out]
                  }
                  frame Disabled {
                  }
                }
                n139 = Index Array(array=w328, index=w322) -> (element=w325:T1)
                n140 = Index Array(array=w326, index=w320) -> (element=w323:string)
                n141 = Bundle By Name(cluster=w325, "Board ID"=w323) -> (w324:T1)
              }
            }
            n142 = call <vilib>:"Add State(s) to Queue__jki_lib_state_machine.vi"("State(s) in Front (\"\")"="Open Newfi Panel", "State(s) in (\"\")"=w317) -> ("States Out"=w316:string)  [unwired: 13 in]
            n143 = Bundle By Name(cluster=w307, "Open Panel"=w313) -> (w314:T10)
          }
          event "Array 3": Value Change {
            # "Row 13-18"
            n144 = event-data() -> ("NewVal"=w344:T1[])  [unwired: 1 in, 5 out]
            n145 = for {
              tunnel: w344 -> [w381] mode=indexing
              tunnel: [w378] -> w348
              tunnel: [w377] -> w350 mode=indexing
              i -> [w378]
              stop <- w379 stop-if-true
              n146 = Unbundle By Name(w381) -> ("Boolean"=w377:bool)
              n147 = Equal?(x=w377, y=TRUE) -> (x = y?=w379:bool)
            }
            n148 = Unbundle By Name(w346) -> ("Open Panel"=w351:T1, "Status Output Locations"=w347:path[], "Connected Board ID's (Newfi)"=w345:string[])
            n149 = Or Array Elements(Boolean array=w350) -> (logical OR=w349:bool)
            n150 = case shown="True" w349 {
              tunnel: w344 -> [_ w367]
              tunnel: w348 -> [_ w362]
              tunnel: [w358 w363] -> w352
              tunnel: w351 -> [w358 _]
              tunnel: w347 -> [_ w366]
              tunnel: w345 -> [_ w365]
              tunnel: 12 ("size(s) 2") -> [_ w361]
              frame False {
              }
              frame True {
                n151 = Add(x=w362, y=w361) -> (x+y=w360:i32)
                n152 = disable-structure shown="Enabled" {
                  disable-tunnel: w360 -> [w369 _]
                  disable-tunnel: w366 -> [w368 _]
                  frame Enabled {
                    n153 = Index Array(array=w368, index=w369) -> (element=w370:path)
                    n154 = Strip Path(path=w370) -> (stripped path=w376:path)  [unwired: 1 out]
                    n155 = Strip Path(path=w376) -> (stripped path=w375:path)  [unwired: 1 out]
                    n156 = Build Path(base path=w375, name or relative path="Newfi.exe") -> (appended path=w373:path)
                    n157 = Path To String(path=w373) -> (string=w372:string)
                    n158 = call <vilib>:"System Exec.vi"("wait until completion? (T)"=FALSE, "command line"=w372) -> ()  [unwired: 6 in, 4 out]
                  }
                  frame Disabled {
                  }
                }
                n159 = Index Array(array=w367, index=w362) -> (element=w364:T1)
                n160 = Index Array(array=w365, index=w360) -> (element=w359:string)
                n161 = Bundle By Name(cluster=w364, "Board ID"=w359) -> (w363:T1)
              }
            }
            n162 = call <vilib>:"Add State(s) to Queue__jki_lib_state_machine.vi"("State(s) in Front (\"\")"="Open Newfi Panel", "State(s) in (\"\")"=w356) -> ("States Out"=w355:string)  [unwired: 13 in]
            n163 = Bundle By Name(cluster=w346, "Open Panel"=w352) -> (w353:T10)
          }
          event "Array 4": Value Change {
            # "19-24"
            n164 = event-data() -> ("NewVal"=w383:T1[])  [unwired: 1 in, 5 out]
            n165 = for {
              tunnel: w383 -> [w420] mode=indexing
              tunnel: [w417] -> w387
              tunnel: [w416] -> w389 mode=indexing
              i -> [w417]
              stop <- w418 stop-if-true
              n166 = Unbundle By Name(w420) -> ("Boolean"=w416:bool)
              n167 = Equal?(x=w416, y=TRUE) -> (x = y?=w418:bool)
            }
            n168 = Unbundle By Name(w385) -> ("Open Panel"=w390:T1, "Status Output Locations"=w386:path[], "Connected Board ID's (Newfi)"=w384:string[])
            n169 = Or Array Elements(Boolean array=w389) -> (logical OR=w388:bool)
            n170 = case shown="True" w388 {
              tunnel: w383 -> [_ w406]
              tunnel: w387 -> [_ w400]
              tunnel: [w397 w402] -> w391
              tunnel: w390 -> [w397 _]
              tunnel: w386 -> [_ w405]
              tunnel: w384 -> [_ w404]
              tunnel: 18 ("size(s) 3") -> [_ w399]
              frame False {
              }
              frame True {
                n171 = Add(x=w400, y=w399) -> (x+y=w398:i32)
                n172 = disable-structure shown="Enabled" {
                  disable-tunnel: w398 -> [w408 _]
                  disable-tunnel: w405 -> [w407 _]
                  frame Enabled {
                    n173 = Index Array(array=w407, index=w408) -> (element=w409:path)
                    n174 = Strip Path(path=w409) -> (stripped path=w415:path)  [unwired: 1 out]
                    n175 = Strip Path(path=w415) -> (stripped path=w414:path)  [unwired: 1 out]
                    n176 = Build Path(base path=w414, name or relative path="Newfi.exe") -> (appended path=w412:path)
                    n177 = Path To String(path=w412) -> (string=w411:string)
                    n178 = call <vilib>:"System Exec.vi"("wait until completion? (T)"=FALSE, "command line"=w411) -> ()  [unwired: 6 in, 4 out]
                  }
                  frame Disabled {
                  }
                }
                n179 = Index Array(array=w406, index=w400) -> (element=w403:T1)
                n180 = Index Array(array=w404, index=w398) -> (element=w401:string)
                n181 = Bundle By Name(cluster=w403, "Board ID"=w401) -> (w402:T1)
              }
            }
            n182 = call <vilib>:"Add State(s) to Queue__jki_lib_state_machine.vi"("State(s) in Front (\"\")"="Open Newfi Panel", "State(s) in (\"\")"=w395) -> ("States Out"=w394:string)  [unwired: 13 in]
            n183 = Bundle By Name(cluster=w385, "Open Panel"=w391) -> (w392:T10)
          }
          event "Settings": Value Change {
            n184 = event-data() -> ()  [unwired: 1 in, 6 out]
            n185 = local write "Tab Control"(enum32{"Page 1", "Page 2"}."Page 2" ("Tab Control")) -> ()
          }
          event "Back Button": Value Change {
            n186 = event-data() -> ()  [unwired: 1 in, 6 out]
            n187 = local write "Tab Control"(enum32{"Page 1", "Page 2"}."Page 1" ("Tab Control")) -> ()
          }
          event Panel Close? {
            n188 = event-data() -> ()  [unwired: 1 in, 1 out]
            n189 = event-data("Discard?"=TRUE) -> ()  [unwired: 1 in, 1 out]
            n190 = call <vilib>:"Add State(s) to Queue__jki_lib_state_machine.vi"("State(s) in Front (\"\")"="Macro: Exit", "State(s) in (\"\")"=w434) -> ("States Out"=w433:string)  [unwired: 13 in]
          }
        }
      }
      frame "---------- Core ----------" {
        # "Do not put any code in this frame.\n(it is a separator no-op)"
        n191 = call <vilib>:"Add State(s) to Queue__jki_lib_state_machine.vi"("State(s) in (\"\")"=w438) -> ("States Out"=w437:string)  [unwired: 14 in]
      }
      frame Default {
        w448 = 42 items=["No error", "Argument error", "Memory is full", "Out of zone", "End of file", "File already open", "Generic file I/O error", "File not found", "File permission error", "Disk is full", "Duplicate path", "Too many files open", "System feature not enabled", "Resource file not found", "Cannot add resource", "Resource not found", "Image not found", "Image memory error", "Pen does not exist", "Config type invalid", "Config token not found", "Config parse error", "Config memory error", "Bad external code format", "Bad external code offset", "External code not present", "Null window", "Destroy window error", "Null menu", "Print aborted", "Bad print record", "Print driver error", "Windows error during printing", "Memory error during printing", "Print dialog error", "Generic print error", "Invalid device refnum", "Device not found", "Device parameter error", "Device unit error", "Cannot open device", "Device call aborted", "Generic error", "Cancelled by user", "Object ID too low", "Object ID too high", "Object not in heap", "Unknown heap", "Unknown object (invalid DefProc)", "Unknown object (DefProc not in table)", "Message out of range", "Invalid (null) method", "Unknown message", "Manager call not supported", "Bad address", "Network operation in progress", "Network operation timed out", "Connection is busy", "Network attribute not supported", "Network error", "Address in use", "System out of memory", "Connection aborted", "Connection refused", "Not connected", "Already connected", "Connection closed", "Initialization error (interapplication manager)", "Bad occurrence", "Wait on unbound occurrence handler", "Occurrence queue overflow", "Datalog type conflict", "Unused", "Unrecognized type (interapplication manager)", "Memory corrupt", "Failed to make temporary DLL", "Old CIN version", "Drag socket not found", "Failed to load drop-object", "Failed to register OLE object", "Failed to release OLE object", "Format specifier type mismatch", "Unknown format specifier", "Too few format specifiers", "Too many format specifiers", "Scan failed", "Newer CIN version", "Error converting to variant", "Runtime menu error", "Password tampered", "Variant attribute not found", "Incompatible variant data type", "Event data is not available", "Event Store is not present", "Occurrence is not found", "Event Queue is not created", "Event info is not available", "Refnum passed is NULL", "Error retrieving Class GUID", "Error retrieving CoClass GUID", "Error retrieving TypeLib GUID.", "Bad built application magic bytes.", "Specific driver is different from the specific driver associated with the Logical Name.", "There is no session opened to the class driver.", "Max Error", "MAX - Error with config objects", "MAX - Error loading configuration", "MAX - Group not supported"]
        # "Current State"
        # "Handle mistyped state name (developer tool)"
        n192 = Format Into String(format string="Software Exception: Unhandled State \"%s\"." ("message"), error in=w444, w439) -> (resulting string=w447:string, error out=w446:errorcluster)  [unwired: 1 in]
        n193 = call <vilib>:"Error Cluster From Error Code.vi"("show call chain? (False)"=TRUE, "error in (no error)"=w446, "error message (\"\")"=w447, "error code (0)"=w448) -> ("error out"=w445:errorcluster)  [unwired: 5 in]
        n194 = call <vilib>:"Add State(s) to Queue__jki_lib_state_machine.vi"("State(s) in (\"\")"=w443) -> ("States Out"=w442:string)  [unwired: 14 in]
      }
      frame "Initialize Core Data" {
        # "originally closed?"
        # "exe?"
        # "If panel starts closed or is an EXE, then close it when we exit"
        n195 = property class="VI"() -> ("Front Panel.Open"=w457:bool)  [unwired: 2 in, 2 out]
        n196 = property class="App"() -> ("App.Kind"=w456:T7)  [unwired: 2 in, 2 out]
        n197 = control-ref of="Current VI Reference"() -> (w450:refnum<vi>)
        n198 = Not(x=w457) -> (.not. x?=w454:bool)
        n199 = Equal?(x=w456, y=T7."Run Time System" ("Application:Kind")) -> (x = y?=w453:bool)
        n200 = Or(x=w454, y=w453) -> (x .or. y?=w451:bool)
        n201 = Bundle By Name(cluster=w452, "Core.Current VI Reference"=w450, "Core.Close Panel on Exit?"=w451) -> (w459:T10)
        n202 = call <vilib>:"Add State(s) to Queue__jki_lib_state_machine.vi"("State(s) in (\"\")"=w461) -> ("States Out"=w460:string)  [unwired: 14 in]
      }
      frame "Error Handler" {
        # "Unhandled Error -- Display it"
        # "Handle any errors here.\nYou can also output any states to clean-up after errors occur"
        # "Clear error"
        n203 = call <vilib>:"General Error Handler.vi"("error in (no error)"=w463) -> ()  [unwired: 10 in, 5 out]
        n204 = call <vilib>:"Add State(s) to Queue__jki_lib_state_machine.vi"("State(s) in Front (\"\")"="/* Post Error States", "State(s) in (\"\")"=w467) -> ("States Out"=w466:string)  [unwired: 13 in]
      }
      frame "Exit" {
        n205 = call <vilib>:"Add State(s) to Queue__jki_lib_state_machine.vi"("State(s) in (\"\")"=w472) -> ("States Out"=w471:string)  [unwired: 14 in]
      }
      frame "---------- Data ----------" {
        # "Do not put any code in this frame.\n(It is a separator no-op. You can make a copy of this frame to create a new Data frame)"
        n206 = call <vilib>:"Add State(s) to Queue__jki_lib_state_machine.vi"("State(s) in (\"\")"=w476) -> ("States Out"=w475:string)  [unwired: 14 in]
      }
      frame "Data: Initialize" {
        n207 = Bundle("Core"=T8 {"Current VI Reference"=refnum, "Close Panel on Exit?"=FALSE}, "Array"="Array", "Array 2"="Array 2", "Status Output Locations"="Status Output Locations", "Open Panel"="Open Panel", "Array 3"="Array 3", "Array 4"="Array 4", "Board Index"="Board Index", "Connected Board ID's (Newfi)"="Connected Board ID's (Newfi)", "Agilent Channels"="", "Start DAQ Loop"="Start DAQ Loop", "Log Debug"=string[] [], "Log Inv & MC"=string[] [], "Station IDs"=string[] [], "Last Save Time"="%H") -> (w493:T10)  [unwired: 1 in]
        n208 = call <vilib>:"Add State(s) to Queue__jki_lib_state_machine.vi"("State(s) in (\"\")"=w495) -> ("States Out"=w494:string)  [unwired: 14 in]
      }
      frame "Read Configuration File" {
        # "Open VISA Session"
        n209 = call-poly <vilib>:"Read From Spreadsheet File.vi"("file path (dialog if empty)"="Configuration Path") -> ("all rows"=w528:string[][])  [unwired: 6 in, 4 out]
        n210 = call-poly <vilib>:"Read From Spreadsheet File.vi"("delimiter (\\t)"="," ("delimiter (\\t)"), "file path (dialog if empty)"="Station and Board IDs") -> ("all rows"=w502:string[][])  [unwired: 5 in, 4 out]
        n211 = Delete From Array(array=w502, index (row)=0) -> (deleted portion=w499:string[], array with subset deleted=w500:string[][])  [unwired: 2 in]
        n212 = Index Array(array=w499, index=1) -> (element=w497:string)
        n213 = Index Array(array=w528, index (col)=0 ("disabled index (col)")) -> (element=w523:string[])  [unwired: 1 in]
        n214 = VISA Open(VISA resource name=w497) -> (VISA resource name=w496:refnum<visa-resource-name>)  [unwired: 4 in, 1 out]
        n215 = for {
          tunnel: w523 -> [w537] mode=indexing
          tunnel: [w536] -> w521 mode=indexing
          n216 = String To Path(string=w537) -> (path=w536:path)
        }
        n217 = Index Array(array=w500, index (col)=1 ("disabled index (col)")) -> (element=w517:string[])  [unwired: 1 in]
        n218 = local write "Agilent"(w496) -> ()
        n219 = Index Array(array=w500, index (col)=2 ("disabled index (col)")) -> (element=w513:string[])  [unwired: 1 in]
        n220 = for {
          tunnel: w517 -> [_] mode=indexing
          tunnel: [w535] -> w516 mode=indexing
          tunnel: w513 -> [w533] mode=indexing
          shift-right: [w532] -> w512
          shift-left: "" -> [w534]
          i -> [w535]
          n221 = Concatenate Strings(w534, w533, "," ("string")) -> (w532:string)
        }
        "Board Index." <- w516
        n222 = Index Array(array=w500, index (col)=0 ("disabled index (col)")) -> (element=w503:string[])  [unwired: 1 in]
        n223 = property on="Status Output Locations" class="Arr (strict)"("Value"=w521) -> ()  [unwired: 2 in, 2 out]
        n224 = call <vilib>:"Trim Whitespace.vi"("string"=w512) -> ("trimmed string"=w511:string)  [unwired: 1 in]
        n225 = String Length(string=w511) -> (length=w507:i32)
        n226 = Decrement(x=w507) -> (x-1=w508:i32)
        n227 = Search and Replace String(input string=w511, search string="," ("string"), replace string="", offset=w508) -> (result string=w506:string)  [unwired: 4 in, 3 out]
        n228 = call <vilib>:"Trim Whitespace.vi"("string"=w506) -> ("trimmed string"=w505:string)  [unwired: 1 in]
        "Agilent Channels DAQ" <- w505
        n229 = Bundle By Name(cluster=w525, "Status Output Locations"=w521, "Connected Board ID's (Newfi)"=w517, "Board Index"=w516, "Agilent Channels"=w505, "Station IDs"=w503) -> (w524:T10)
        n230 = call <vilib>:"Add State(s) to Queue__jki_lib_state_machine.vi"("State(s) in (\"\")"=w526) -> ("States Out"=w530:string)  [unwired: 14 in]
      }
      frame "Show Station Labels" {
        n231 = Unbundle By Name(w543) -> ("Station IDs"=w553:string[], "Array"=w551:T1[], "Array 2"=w550:T1[], "Array 3"=w549:T1[], "Array 4"=w548:T1[])
        n232 = call "Extract Rows.vi"("String"=w553, "Enum"=enum16{"0-6", "6-6", "6-12", "6-18"}."0-6") -> ("String Output"=w547:string[])  [unwired: 7 in, 2 out]
        n233 = call "Extract Rows.vi"("String"=w553, "Enum"=enum16{"0-6", "6-6", "6-12", "6-18"}."6-6") -> ("String Output"=w546:string[])  [unwired: 7 in, 2 out]
        n234 = call "Extract Rows.vi"("String"=w553, "Enum"=enum16{"0-6", "6-6", "6-12", "6-18"}."6-12") -> ("String Output"=w545:string[])  [unwired: 7 in, 2 out]
        n235 = call "Extract Rows.vi"("String"=w553, "Enum"=enum16{"0-6", "6-6", "6-12", "6-18"}."6-18") -> ("String Output"=w544:string[])  [unwired: 7 in, 2 out]
        n236 = for {
          tunnel: w551 -> [w571] mode=indexing
          tunnel: w550 -> [w570] mode=indexing
          tunnel: w549 -> [w569] mode=indexing
          tunnel: w548 -> [w568] mode=indexing
          tunnel: w547 -> [w567] mode=indexing
          tunnel: w546 -> [w566] mode=indexing
          tunnel: w545 -> [w565] mode=indexing
          tunnel: w544 -> [w564] mode=indexing
          tunnel: [w563] -> w541 mode=indexing
          tunnel: [w562] -> w540 mode=indexing
          tunnel: [w561] -> w539 mode=indexing
          tunnel: [w560] -> w538 mode=indexing
          n237 = Bundle By Name(cluster=w571, "Station Label"=w567) -> (w563:T1)
          n238 = Bundle By Name(cluster=w570, "Station Label"=w566) -> (w562:T1)
          n239 = Bundle By Name(cluster=w569, "Station Label"=w565) -> (w561:T1)
          n240 = Bundle By Name(cluster=w568, "Station Label"=w564) -> (w560:T1)
        }
        n241 = Bundle By Name(cluster=w543, "Array"=w541, "Array 2"=w540, "Array 3"=w539, "Array 4"=w538) -> (w542:T10)
        n242 = call <vilib>:"Add State(s) to Queue__jki_lib_state_machine.vi"("State(s) in (\"\")"=w558) -> ("States Out"=w559:string)  [unwired: 14 in]
      }
      frame "Data: Cleanup" {
        n243 = Unbundle By Name(w572) -> ("Core.Current VI Reference"=w575:refnum<vi>)
        n244 = Close Reference(reference=w575, error in (no error)=w574) -> (error out=w573:errorcluster)
        n245 = call <vilib>:"Add State(s) to Queue__jki_lib_state_machine.vi"("State(s) in (\"\")"=w577) -> ("States Out"=w576:string)  [unwired: 14 in]
      }
      frame "---------- UI ----------" {
        # "Do not put any code in this frame.\n(It is a separator no-op. You can make a copy of this frame to create a new UI frame)"
        n246 = call <vilib>:"Add State(s) to Queue__jki_lib_state_machine.vi"("State(s) in (\"\")"=w581) -> ("States Out"=w580:string)  [unwired: 14 in]
      }
      frame "UI: Initialize" {
        w582 = T1[] [{"Serial Number"="", "Day Cycle Count"=0, "Station Label"="", "Status Color"=0, "Current Run Start Time"=0.0, "Audit Alert"=FALSE, "Washer Details"={"Cycle Count"="", "Status"="", "Notes"="", "Lab ID"="", "Total Time On"="", "TR Number"=""}, "Board ID"="", "Boolean"=FALSE, "RPM"=0, "Current"=0.0, "Current Path"=path "", "Saving"=FALSE, "Unit Type"=0}, {"Serial Number"="", "Day Cycle Count"=0, "Station Label"="", "Status Color"=0, "Current Run Start Time"=0.0, "Audit Alert"=FALSE, "Washer Details"={"Cycle Count"="", "Status"="", "Notes"="", "Lab ID"="", "Total Time On"="", "TR Number"=""}, "Board ID"="", "Boolean"=FALSE, "RPM"=0, "Current"=0.0, "Current Path"=path "", "Saving"=FALSE, "Unit Type"=0}, {"Serial Number"="", "Day Cycle Count"=0, "Station Label"="", "Status Color"=0, "Current Run Start Time"=0.0, "Audit Alert"=FALSE, "Washer Details"={"Cycle Count"="", "Status"="", "Notes"="", "Lab ID"="", "Total Time On"="", "TR Number"=""}, "Board ID"="", "Boolean"=FALSE, "RPM"=0, "Current"=0.0, "Current Path"=path "", "Saving"=FALSE, "Unit Type"=0}, {"Serial Number"="", "Day Cycle Count"=0, "Station Label"="", "Status Color"=0, "Current Run Start Time"=0.0, "Audit Alert"=FALSE, "Washer Details"={"Cycle Count"="", "Status"="", "Notes"="", "Lab ID"="", "Total Time On"="", "TR Number"=""}, "Board ID"="", "Boolean"=FALSE, "RPM"=0, "Current"=0.0, "Current Path"=path "", "Saving"=FALSE, "Unit Type"=0}, {"Serial Number"="", "Day Cycle Count"=0, "Station Label"="", "Status Color"=0, "Current Run Start Time"=0.0, "Audit Alert"=FALSE, "Washer Details"={"Cycle Count"="", "Status"="", "Notes"="", "Lab ID"="", "Total Time On"="", "TR Number"=""}, "Board ID"="", "Boolean"=FALSE, "RPM"=0, "Current"=0.0, "Current Path"=path "", "Saving"=FALSE, "Unit Type"=0}, {"Serial Number"="", "Day Cycle Count"=0, "Station Label"="", "Status Color"=0, "Current Run Start Time"=0.0, "Audit Alert"=FALSE, "Washer Details"={"Cycle Count"="", "Status"="", "Notes"="", "Lab ID"="", "Total Time On"="", "TR Number"=""}, "Board ID"="", "Boolean"=FALSE, "RPM"=0, "Current"=0.0, "Current Path"=path "", "Saving"=FALSE, "Unit Type"=0}] ("Array")
        n247 = property on="Array 3" class="Arr (strict)"("Value"=w582) -> ()  [unwired: 2 in, 2 out]
        n248 = property on="Array 4" class="Arr (strict)"("Value"=w582) -> ()  [unwired: 2 in, 2 out]
        n249 = property on="Array" class="Arr (strict)"("Value"=w582) -> ()  [unwired: 2 in, 2 out]
        n250 = property on="Array 2" class="Arr (strict)"("Value"=w582) -> ()  [unwired: 2 in, 2 out]
        n251 = Bundle By Name(cluster=w584, "Array"=w582, "Array 2"=w582, "Array 3"=w582, "Array 4"=w582) -> (w583:T10)
        n252 = call <vilib>:"Add State(s) to Queue__jki_lib_state_machine.vi"("State(s) in (\"\")"=w587) -> ("States Out"=w586:string)  [unwired: 14 in]
      }
      frame "UI: Cursor Set" {
        # "Argument"
        n253 = case shown="\"Idle\", Default" w588 {
          tunnel: w590 -> [w595 w597]
          tunnel: [w594 w596] -> w589
          frame "Idle", Default {
            n254 = call <vilib>:"Unset Busy.vi"("error in (no error)"=w595) -> ("error out"=w594:errorcluster)  [unwired: 10 in]
          }
          frame "Busy" {
            n255 = call <vilib>:"Set Busy.vi"("error in (no error)"=w597) -> ("error out"=w596:errorcluster)  [unwired: 9 in, 1 out]
          }
        }
        n256 = call <vilib>:"Add State(s) to Queue__jki_lib_state_machine.vi"("State(s) in (\"\")"=w593) -> ("States Out"=w592:string)  [unwired: 14 in]
      }
      frame "UI: Front Panel State" {
        # "Argument"
        n257 = Unbundle By Name(w601) -> ("Core.Current VI Reference"=w600:refnum<vi>)
        n258 = case shown="\"Open\", Default" w599 {
          tunnel: w603 -> [w609 w622]
          tunnel: [w611 w623] -> w602
          tunnel: w600 -> [w610 w620]
          frame "Open", Default {
            n259 = property class="VI"(reference=w610, error in=w609) -> (reference out=w607:refnum<vi>, error out=w608:errorcluster, "Front Panel.Open"=w606:bool)
            n260 = case shown="True" w606 {
              tunnel: [w612 w615] -> w611
              tunnel: w608 -> [w612 w614]
              tunnel: w607 -> [_ w613]
              frame False {
              }
              frame True {
                n261 = invoke class="VI" method="FP.Open"(reference=w613, error in=w614, "Activate"=TRUE, "State"=T9."Maximized") -> (error out=w615:errorcluster)  [unwired: 1 in, 4 out]
              }
            }
          }
          frame "Close" {
            n262 = property class="VI"(reference=w620, error in=w622) -> (reference out=w619:refnum<vi>, error out=w621:errorcluster, "Front Panel.Open"=w618:bool)
            n263 = case shown="True" w618 {
              tunnel: [w624 w627] -> w623
              tunnel: w621 -> [w624 w626]
              tunnel: w619 -> [_ w625]
              frame False {
              }
              frame True {
                n264 = invoke class="VI" method="FP.Close"(reference=w625, error in=w626) -> (error out=w627:errorcluster)  [unwired: 1 in, 2 out]
              }
            }
          }
        }
        n265 = local write "Start DAQ Loop"(TRUE ("Start DAQ Loop")) -> ()
        n266 = call <vilib>:"Add State(s) to Queue__jki_lib_state_machine.vi"("State(s) in (\"\")"=w605) -> ("States Out"=w604:string)  [unwired: 14 in]
      }
      frame "---------- Macro ----------" {
        # "Do not put any code in this frame.\n(It is a separator no-op. You can make a copy of this frame to create a new Macro frame)"
        n267 = call <vilib>:"Add State(s) to Queue__jki_lib_state_machine.vi"("State(s) in (\"\")"=w631) -> ("States Out"=w630:string)  [unwired: 14 in]
      }
      frame "Macro: Initialize" {
        w632 = "Data: Initialize\nRead Configuration File\nInitialize Core Data\nUI: Initialize\nShow Station Labels\nUI: Front Panel State >> Open"  # Data: Initialize Read Configuration File Initialize Core Data UI: Initialize Show Station Labels UI: Front Panel State >> Open
        n268 = call <vilib>:"Add State(s) to Queue__jki_lib_state_machine.vi"("State(s) in Front (\"\")"=w632, "State(s) in (\"\")"=w636) -> ("States Out"=w635:string)  [unwired: 13 in]
      }
      frame "Macro: Exit" {
        n269 = Unbundle By Name(w643) -> ("Core.Close Panel on Exit?"=w642:bool)
        n270 = Select(t="UI: Front Panel State >> Close", s=w642, f="") -> (s? t:f=w639:string)
        n271 = call <vilib>:"Add State(s) to Queue__jki_lib_state_machine.vi"("State(s) in (\"\")"=w639, "State(s) at Back (\"\")"="Data: Cleanup\nExit") -> ("States Out"=w637:string)  [unwired: 13 in]
        n272 = call <vilib>:"Add State(s) to Queue__jki_lib_state_machine.vi"("State(s) in Front (\"\")"=w637, "State(s) in (\"\")"=w646) -> ("States Out"=w645:string)  [unwired: 13 in]
      }
      frame "---------- New Category ----------" {
        # "Template Separator\n(You can make a copy of, or modify, this frame)"
        n273 = call <vilib>:"Add State(s) to Queue__jki_lib_state_machine.vi"("State(s) in (\"\")"=w650) -> ("States Out"=w649:string)  [unwired: 14 in]
      }
      frame "Update Status" {
        w658 = enum16{"0-6", "6-6", "6-12", "6-18"}."6-18" ("Enum")
        w663 = enum16{"0-6", "6-6", "6-12", "6-18"}."6-12" ("Enum")
        w668 = enum16{"0-6", "6-6", "6-12", "6-18"}."6-6" ("Enum")
        w666 = enum16{"0-6", "6-6", "6-12", "6-18"}."0-6" ("Enum")
        n274 = Unbundle By Name(w683) -> ("Array"=w681:T1[], "Array 2"=w679:T1[], "Array 3"=w677:T1[], "Array 4"=w675:T1[], "Board Index"=w657:i32[])
        n275 = local read "Save Array"() -> (w652:bool[])
        n276 = local read "Current"() -> (w651:dbl[])
        n277 = call "Extract Rows.vi"("Enum"=w663, "Board Index"=w657) -> ("Array"=w665:dbl[])  [unwired: 7 in, 2 out]
        n278 = call "Extract Rows.vi"("Enum"=w666, "Board Index"=w657) -> ("Array"=w673:dbl[])  [unwired: 7 in, 2 out]
        n279 = call "Extract Rows.vi"("Saving"=w652, "Enum"=w666, "Board Index"=w651) -> ("Boolean Array"=w653:bool[], "Array"=w671:dbl[])  [unwired: 6 in, 1 out]
        n280 = call "Extract Rows.vi"("Enum"=w668, "Board Index"=w657) -> ("Array"=w670:dbl[])  [unwired: 7 in, 2 out]
        n281 = call "Extract Rows.vi"("Saving"=w652, "Enum"=w668, "Board Index"=w651) -> ("Boolean Array"=w654:bool[], "Array"=w667:dbl[])  [unwired: 6 in, 1 out]
        n282 = call "Extract Rows.vi"("Saving"=w652, "Enum"=w663, "Board Index"=w651) -> ("Boolean Array"=w655:bool[], "Array"=w662:dbl[])  [unwired: 6 in, 1 out]
        n283 = call "Extract Rows.vi"("Enum"=w658, "Board Index"=w657) -> ("Array"=w661:dbl[])  [unwired: 7 in, 2 out]
        n284 = call "Extract Rows.vi"("Saving"=w652, "Enum"=w658, "Board Index"=w651) -> ("Boolean Array"=w656:bool[], "Array"=w659:dbl[])  [unwired: 6 in, 1 out]
        n285 = To Long Integer(number=w673) -> (32bit integer=w672:i32[])
        n286 = To Long Integer(number=w665) -> (32bit integer=w664:i32[])
        n287 = To Long Integer(number=w670) -> (32bit integer=w669:i32[])
        n288 = To Long Integer(number=w661) -> (32bit integer=w660:i32[])
        n289 = call "Extract Newtwork Variable.vi"("Saving"=w653, "Current"=w671, "Array in"=w672, "Array 3"=w681) -> ("Array out"=w680:T1[])  [unwired: 7 in]
        n290 = call "Extract Newtwork Variable.vi"("Saving"=w654, "Current"=w667, "Array in"=w669, "Array 3"=w679) -> ("Array out"=w678:T1[])  [unwired: 7 in]
        n291 = call "Extract Newtwork Variable.vi"("Saving"=w655, "Current"=w662, "Array in"=w664, "Array 3"=w677) -> ("Array out"=w676:T1[])  [unwired: 7 in]
        n292 = call "Extract Newtwork Variable.vi"("Saving"=w656, "Current"=w659, "Array in"=w660, "Array 3"=w675) -> ("Array out"=w674:T1[])  [unwired: 7 in]
        n293 = property on="Array" class="Arr (strict)"("Value"=w680) -> ()  [unwired: 2 in, 2 out]
        n294 = property on="Array 2" class="Arr (strict)"("Value"=w678) -> ()  [unwired: 2 in, 2 out]
        n295 = property on="Array 3" class="Arr (strict)"("Value"=w676) -> ()  [unwired: 2 in, 2 out]
        n296 = property on="Array 4" class="Arr (strict)"("Value"=w674) -> ()  [unwired: 2 in, 2 out]
        n297 = Bundle By Name(cluster=w683, "Array"=w680, "Array 2"=w678, "Array 3"=w676, "Array 4"=w674) -> (w682:T10)
        n298 = call <vilib>:"Add State(s) to Queue__jki_lib_state_machine.vi"("State(s) in (\"\")"=w686) -> ("States Out"=w685:string)  [unwired: 14 in]
      }
      frame "Open Newfi Panel" {
        n299 = Unbundle By Name(w689) -> ("Open Panel.Board ID"=w687:string)
        n300 = shared-variable ".\\Test Lib.lvlib\\Board ID"(w687) -> ()  [unwired: 1 in, 1 out]
        n301 = call <vilib>:"Add State(s) to Queue__jki_lib_state_machine.vi"("State(s) in (\"\")"=w691) -> ("States Out"=w690:string)  [unwired: 14 in]
      }
      frame "Check Robocopy" {
        n302 = Unbundle By Name(w693) -> ()  [unwired: 1 out]
        n303 = call <vilib>:"Add State(s) to Queue__jki_lib_state_machine.vi"("State(s) in (\"\")"=w695) -> ("States Out"=w694:string)  [unwired: 14 in]
      }
    }
    "States Out 2" <- w235
  }
